vi "spectrum_display.vi"(5 "Modulation info":T8 {"Hi channels at low" min=0 step=1; "Low carriers" format="%#_6p"; "High carriers" format="%#_6p"}, 6 "Reset STFT":bool, 7 "Config":T2={"IO params"={"Conversion"={"Rate"=0.0, "In channels"=0, "Out channels"=4}, "Carriers"={"Phase shift"=180.0, "Levels"=[[0.8, 0.8, 0.8], [0.03, 0.03, 0.03]], "Delay samples"=73.15}}, "High rate STFT"={"Win param"=0.0, "Window type"=0, "Win order"=0, "DFT size"=0, "Channels"=[], "Oversample"=0}, "Low rate STFT"={"Win param"=0.0, "Window type"=0, "Win order"=0, "DFT size"=0, "Channels"=[], "Oversample"=0}, "Filtering"={"Hum"={"Frequency"=0.0, "Tc"=0.0, "Limit"=0.0, "FFT filter"=FALSE, "Detrend mode"=enum."Robust linear", "Enable"=FALSE}, "Kalman"={"Process noise"=0.0, "Measure noise"=0.0, "Unlock m noise"=0.0, "Mode"=enum."FFT"}, "Distortion"={"LF cut"=0.0, "Tc"=0.0, "Limit"=0.0, "FFT filter"=FALSE, "Detrend mode"=enum."Robust linear", "Enable"=FALSE}, "Lowpass"={"Frequency"=0.0, "Order"=0, "Enable"=FALSE}, "Impulse"={"Win order"=0, "Locked limit"=0.0, "Locked count"=0, "Threshold Tc"=0.0, "Thresh sigmas"=0.0, "Thresh min"=0.0, "After"=0, "Detrend"=FALSE, "Enable"=FALSE}}} {"Filtering"."Impulse"."Thresh min" format="%#_3p"; "Filtering"."Impulse"."Threshold Tc" format="%#_3p"; "Filtering"."Impulse"."Locked limit" format="%#_3p"; "Filtering"."Impulse"."Thresh sigmas" format="%#_3p"; "Filtering"."Lowpass"."Frequency" format="%#_4p"; "Filtering"."Distortion"."Limit" format="%#_3p"; "Filtering"."Distortion"."LF cut" format="%#_3p"; "Filtering"."Kalman"."Unlock m noise" format="%#_3p"; "Filtering"."Kalman"."Measure noise" format="%#_3p"; "Filtering"."Kalman"."Process noise" format="%#_3p"; "Filtering"."Hum"."Limit" format="%#_3p"; "Filtering"."Hum"."Frequency" format="%#_4p"; "Low rate STFT"."Oversample" min=1 step=1; "Low rate STFT"."Channels" min=0 step=1; "Low rate STFT"."DFT size" min=1 step=1; "Low rate STFT"."Window type" items=["Rectangle"=0, "Hanning"=1, "Hamming"=2, "Blackman-Harris"=3, "Exact Blackman"=4, "Blackman"=5, "Flat Top"=6, "4 Term B-Harris "=7, "7 Term B-Harris"=8, "Low Sidelobe"=9, "Blackman Nuttall"=11, "Triangle"=30, "Bartlett-Hanning"=31, "Bohman"=32, "Parzen"=33, "Welch"=34, "Kaiser"=60, "Dolph-Chebyshev"=61, "Gaussian"=62]; "High rate STFT"."Oversample" min=1 step=1; "High rate STFT"."Channels" min=0 step=1; "High rate STFT"."DFT size" min=1 step=1; "High rate STFT"."Window type" items=["Rectangle"=0, "Hanning"=1, "Hamming"=2, "Blackman-Harris"=3, "Exact Blackman"=4, "Blackman"=5, "Flat Top"=6, "4 Term B-Harris "=7, "7 Term B-Harris"=8, "Low Sidelobe"=9, "Blackman Nuttall"=11, "Triangle"=30, "Bartlett-Hanning"=31, "Bohman"=32, "Parzen"=33, "Welch"=34, "Kaiser"=60, "Dolph-Chebyshev"=61, "Gaussian"=62]; "IO params"."Carriers"."Levels" min=0.0 step=0.1; "IO params"."Conversion"."Rate" format="%#_8g"}, 9 "Restart Averaging":bool, 10 "Spectrum parameters":T1={"Window"=enum."7 Term B-Harris", "FFT blocking"=enum."1", "Averaging"=5.0, "Order"=2} {"Order" min=1 max=100; "Averaging" min=0.0 max=1000.0 step=1.0}, 11 "Time domain wavevorms":waveform(dbl)[](array[waveform])) -> (2 "Complex spectrum":waveform(cdb)[](array[waveform]), 3 "dB spectrum":waveform(dbl)[](array[waveform]))   [LabVIEW 2014]
uses:
  modulation_info.ctl
  ilemt_config.ctl
  IO_params.ctl
  stft_params.ctl
  <vilib>/Analysis/4window.llb/windowTd.ctl
  filter_params.ctl
  detrend_mode.ctl
  spectrum_parameters.ctl
  <vilib>/Analysis/NI_AALPro.lvlib
panel:
  out "time-freq sample info":cluster{"time steps":i32, "frequency bins":i32}
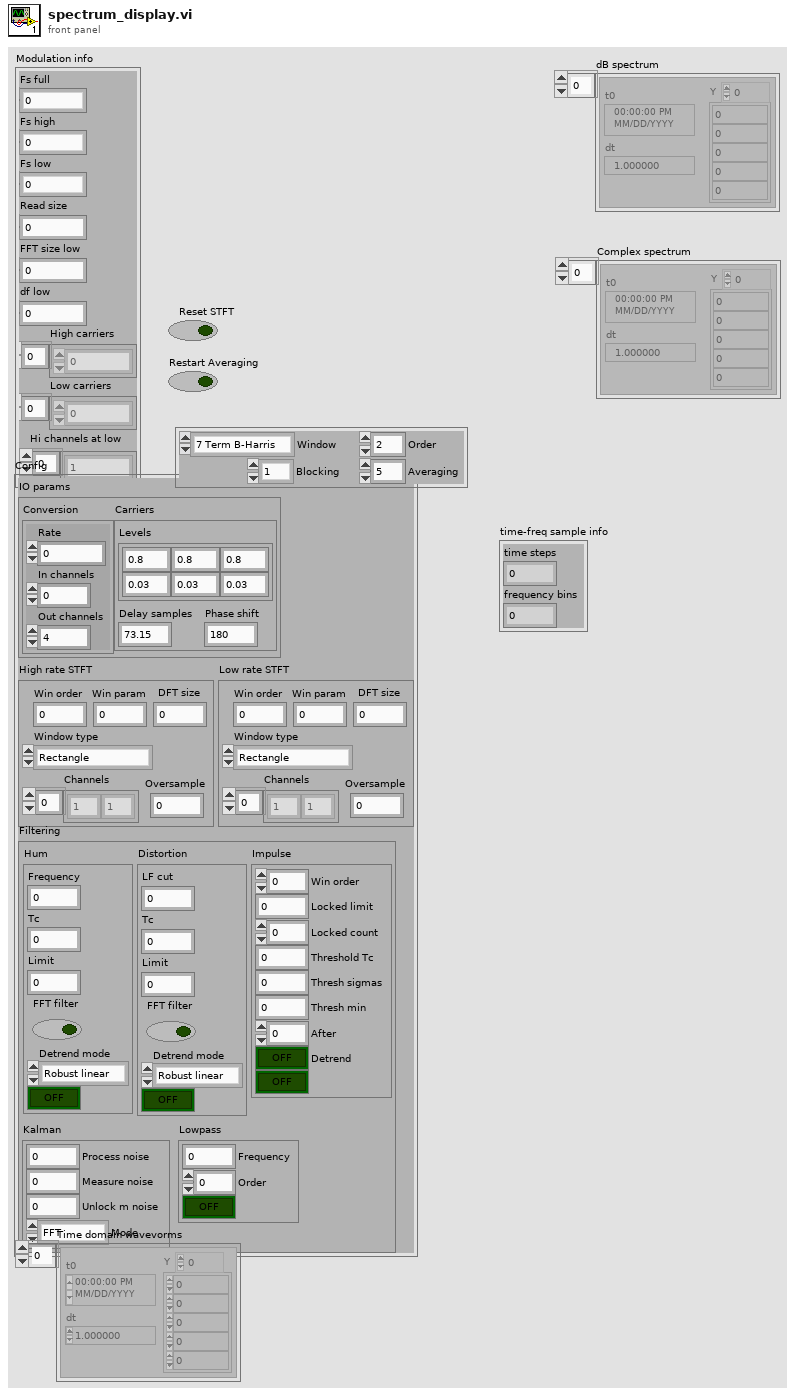
[diagram p1: front panel]
types:
  T1 = typedef "spectrum_parameters.ctl" = cluster{"Window":enum16{"None ", "Hanning", "Hamming", "Blackman-Harris", "Exact Blackman", "Blackman", "Flat Top", "4 Term B-Harris ", "7 Term B-Harris", "Low Sidelobe"}, "FFT blocking":enum16{"1", "2", "4", "8"}, "Averaging":dbl, "Order":u32}
  T2 = typedef "ilemt_config.ctl" = cluster{"IO params":T3, "High rate STFT":T4, "Low rate STFT":T4, "Filtering":T6}
  T3 = typedef "IO_params.ctl" = cluster{"Conversion":cluster{"Rate":dbl, "In channels":u32, "Out channels":u32}, "Carriers":cluster{"Phase shift":dbl, "Levels":dbl[][], "Delay samples":dbl}}
  T4 = typedef "stft_params.ctl" = cluster{"Win param":dbl, "Window type":T5, "Win order":i32, "DFT size":i32, "Channels":i32[], "Oversample":i32}
  T5 = typedef "NI_AALPro.lvlib/windowTd.ctl" = u32
  T6 = typedef "filter_params.ctl" = cluster{"Hum":cluster{"Frequency":dbl, "Tc":dbl, "Limit":dbl, "FFT filter":bool, "Detrend mode":T7, "Enable":bool}, "Kalman":cluster{"Process noise":dbl, "Measure noise":dbl, "Unlock m noise":dbl, "Mode":enum16{"FFT", "KF demod"}}, "Distortion":cluster{"LF cut":dbl, "Tc":dbl, "Limit":dbl, "FFT filter":bool, "Detrend mode":T7, "Enable":bool}, "Lowpass":cluster{"Frequency":dbl, "Order":i32, "Enable":bool}, "Impulse":cluster{"Win order":i32, "Locked limit":dbl, "Locked count":i32, "Threshold Tc":dbl, "Thresh sigmas":dbl, "Thresh min":dbl, "After":i32, "Detrend":bool, "Enable":bool}}
  T7 = typedef "detrend_mode.ctl" = enum16{"Zero mean", "Linear", "Robust linear"}
  T8 = typedef "modulation_info.ctl" = cluster{"Fs full":dbl, "Fs high":dbl, "Fs low":dbl, "Read size":i32, "FFT size low":i32, "df low":dbl, "High carriers":dbl[], "Low carriers":dbl[], "Hi channels at low":i32[]}
  T9 = enum16{"None ", "Hanning", "Hamming", "Blackman-Harris", "Exact Blackman", "Blackman", "Flat Top", "4 Term B-Harris ", "7 Term B-Harris", "Low Sidelobe"}
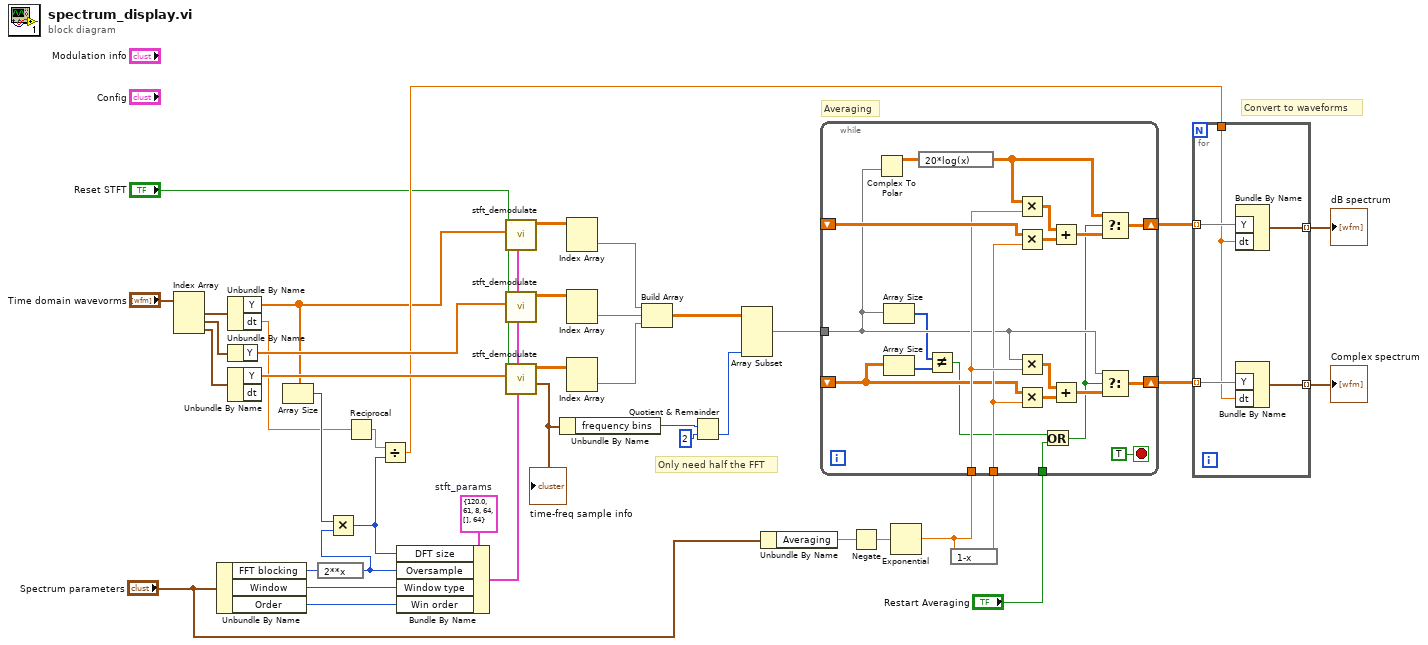
[diagram p0: block diagram]
diagram:
  w12 = T4 {"Win param"=120.0, "Window type"=61, "Win order"=8, "DFT size"=64, "Channels"=[], "Oversample"=64}  # stft_params
  # "Convert to waveforms"
  # "Averaging"
  # "Only need half the FFT"
  n1 = Index Array(array="Time domain wavevorms") -> (element #1=w39:waveform(dbl), element #2=w38:waveform(dbl), element #3=w37:waveform(dbl))  [unwired: 3 in]
  n2 = Unbundle By Name("Spectrum parameters") -> ("FFT blocking"=w8:enum16{"1", "2", "4", "8"}, "Window"=w34:T9, "Order"=w33:u32)
  n3 = Unbundle By Name(w39) -> ("Y"=w2:dbl[], "dt"=w1:dbl)
  n4 = Unbundle By Name(w38) -> ("Y"=w36:dbl[])
  n5 = Unbundle By Name(w37) -> ("Y"=w7:dbl[])  [unwired: 1 out]
  n6 = Array Size(array=w2) -> (size(s)=w11:i32)
  n7 = expression code="2**x"(w8) -> (w5:enum16{"1", "2", "4", "8"})
  n8 = Multiply(x=w11, y=w5) -> (x*y=w6:i32)
  n9 = Reciprocal(x=w1) -> (1/x=w35:dbl)
  n10 = Divide(x=w35, y=w6) -> (x/y=w4:dbl)
  n11 = Bundle By Name(cluster=w12, "DFT size"=w6, "Oversample"=w5, "Window type"=w34, "Win order"=w33) -> (w40:T4)
  n12 = call "stft_demodulate.vi"("STFT params"=w40, "Reset"="Reset STFT", "X"=w2) -> ("STFT"=w32:cdb[][])  [unwired: 6 in, 2 out]
  n13 = call "stft_demodulate.vi"("STFT params"=w40, "Reset"="Reset STFT", "X"=w36) -> ("STFT"=w31:cdb[][])  [unwired: 6 in, 2 out]
  n14 = call "stft_demodulate.vi"("STFT params"=w40, "Reset"="Reset STFT", "X"=w7) -> ("time-freq sample info"=w20:cluster{"time steps":i32, "frequency bins":i32}, "STFT"=w30:cdb[][])  [unwired: 6 in, 1 out]
  "time-freq sample info" <- w20
  n15 = Unbundle By Name(w20) -> ("frequency bins"=w19:i32)
  n16 = Index Array(array=w32) -> (element=w29:cdb[])  [unwired: 2 in]
  n17 = Index Array(array=w31) -> (element=w28:cdb[])  [unwired: 2 in]
  n18 = Index Array(array=w30) -> (element=w27:cdb[])  [unwired: 2 in]
  n19 = Build Array(w29, w28, w27) -> (w21:cdb[][])
  n20 = Quotient & Remainder(x=w19, y=2) -> (floor(x/y)=w18:i32)  [unwired: 1 out]
  n21 = Array Subset(array=w21, length (col)=w18) -> (w17:cdb[][])  [unwired: 3 in]
  n22 = Unbundle By Name("Spectrum parameters") -> ("Averaging"=w26:dbl)
  n23 = Negate(x=w26) -> (-x=w25:dbl)
  n24 = Exponential(1:w25) -> (0:w24:dbl)
  n25 = expression code="1-x"(w24) -> (w23:dbl)
  n26 = while {
    tunnel: w24 -> [w50]
    tunnel: w23 -> [w49]
    shift-right: [w61] -> w16
    shift-left: _ -> [w55]
    tunnel: "Restart Averaging" -> [w43]
    tunnel: w17 -> [w48]
    shift-right: [w51] -> w15
    shift-left: _ -> [w47]
    stop <- TRUE stop-if-true
    n27 = Complex To Polar(r * e^(i*theta)=w48) -> (r=w62:dbl[][])  [unwired: 1 out]
    n28 = Array Size(array=w48) -> (size(s)=w45:i32[])
    n29 = Array Size(array=w47) -> (size(s)=w46:i32[])
    n30 = expression code="20*log(x)"(w62) -> (w58:dbl[][])
    n31 = Not Equal?(x=w45, y=w46) -> (x != y?=w44:bool)
    n32 = Multiply(x=w58, y=w50) -> (x*y=w60:dbl[][])
    n33 = Multiply(x=w55, y=w49) -> (x*y=w59:dbl[][])
    n34 = Multiply(x=w48, y=w50) -> (x*y=w52:cdb[][])
    n35 = Multiply(x=w47, y=w49) -> (x*y=w53:cdb[][])
    n36 = Or(x=w44, y=w43) -> (x .or. y?=w42:bool)
    n37 = Add(x=w60, y=w59) -> (x+y=w57:dbl[][])
    n38 = Add(x=w52, y=w53) -> (x+y=w54:cdb[][])
    n39 = Select(t=w58, s=w42, f=w57) -> (s? t:f=w61:dbl[][])
    n40 = Select(t=w48, s=w42, f=w54) -> (s? t:f=w51:cdb[][])
  }
  n41 = for {
    tunnel: w16 -> [w67] mode=indexing
    tunnel: w15 -> [w65] mode=indexing
    tunnel: w4 -> [w63]
    tunnel: [w66] -> w14 mode=indexing
    tunnel: [w64] -> w13 mode=indexing
    n42 = Bundle By Name("Y"=w67, "dt"=w63) -> (w66:waveform(dbl))  [unwired: 1 in]
    n43 = Bundle By Name("Y"=w65, "dt"=w63) -> (w64:waveform(cdb))  [unwired: 1 in]
  }
  "Complex spectrum" <- w13
  "dB spectrum" <- w14
